vi "Build Msg Buffer.vi"(10 "View Msgs":bool, 11 "Message":string) -> (3 "String":string)   [LabVIEW 2015]
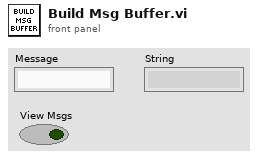
[diagram p1: front panel]
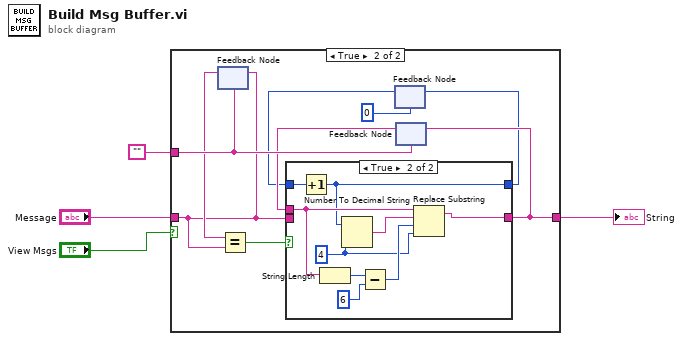
[diagram p0: block diagram]
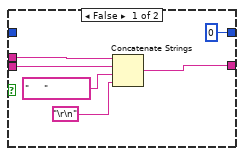
[diagram p3: hidden frame]
diagram:
  n1 = case shown="True" "View Msgs" {
    tunnel: "Message" -> [_ w10]
    tunnel: [_ w13] -> w4
    tunnel: "" -> [_ w12]
    frame False {
    }
    frame True {
      n2 = feedback-in #1(w10) -> ()
      n3 = feedback #1(w12) -> (w11:string)
      n4 = Equal?(x=w11, y=w10) -> (x = y?=w8:bool)
      n5 = feedback #2(u32 0) -> (w6:u32)
      n6 = feedback #3(w12) -> (w9:string)
      n7 = case shown="True" w8 {
        tunnel: [w19 w21] -> w13
        tunnel: w10 -> [w18 _]
        tunnel: w9 -> [w16 w28]
        tunnel: w6 -> [_ w26]
        tunnel: [u32 0 w24] -> w5
        frame False {
          n8 = Concatenate Strings(w16, w18, "     ", "\r\n") -> (w19:string)
        }
        frame True {
          w20 = i16 4
          n9 = Increment(x=w26) -> (x+1=w24:u32)
          n10 = String Length(string=w28) -> (length=w25:i32)
          n11 = Number To Decimal String(number=w24, width (-)=w20) -> (decimal integer string=w23:string)
          n12 = Subtract(x=w25, y=6) -> (x-y=w27:i32)
          n13 = Replace Substring(2:w20, 3:w27, 4:w23, 5:w28) -> (1:w21:string)  [unwired: 1 out]
        }
      }
      n14 = feedback-in #2(w5) -> ()
      n15 = feedback-in #3(w13) -> ()
    }
  }
  "String" <- w4
